vi "Configure ADXL345.vi"(8 "error in":errorcluster, 10 "Port":i8, 11 "FPGA VI Reference":T1) -> (0 "error out":errorcluster, 3 "FPGA VI Reference Out":T1)   [LabVIEW 2014]
uses:
  Controls/FPGA Reference.ctl
  Controls/SPI Configuration Cluster.ctl
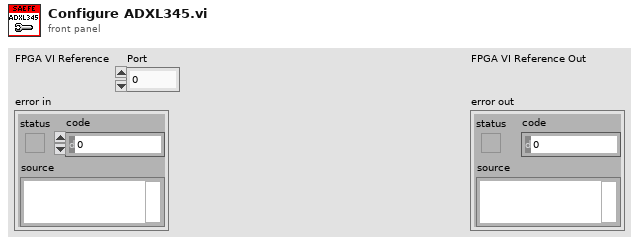
[diagram p1: front panel]
types:
  T1 = typedef "FPGA Reference.ctl" = refnum<k20>
  T2 = typedef "SPI Configuration Cluster.ctl" = cluster{"CS":u8, "Clock Rate (Hz)":dbl, "Clock Mode":u8, "CS Active State":bool}
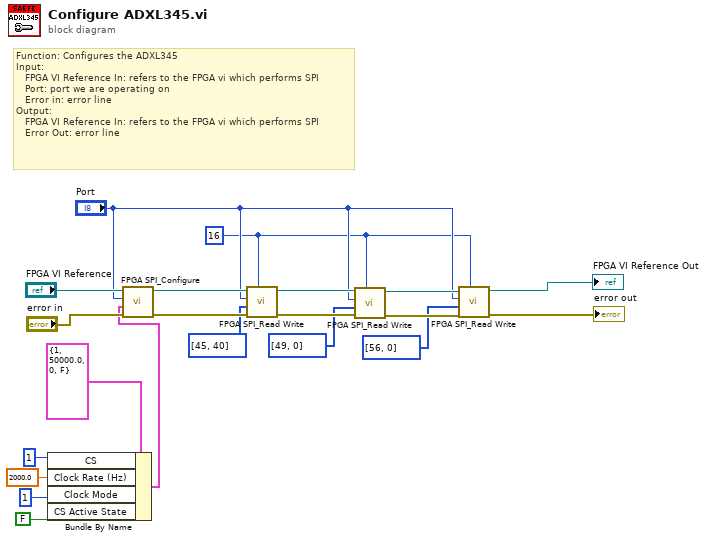
[diagram p0: block diagram]
diagram:
  w3 = u16 16 ("Total Bits")
  # "Function: Configures the ADXL345\nInput:\n   FPGA VI Reference In: refers to the FPGA vi which performs SPI\n   Port: port we are operating on\n   Error in: error line\nOutput:\n   FPGA VI Reference In: refers to the FPGA vi which performs SPI\n   Error Out: error line"
  n1 = Bundle By Name(cluster=T2 {"CS"=1, "Clock Rate (Hz)"=50000.0, "Clock Mode"=0, "CS Active State"=FALSE} ("Configuration Cluster"), "CS"=u8 1, "Clock Rate (Hz)"=2000.0, "Clock Mode"=u8 1, "CS Active State"=FALSE) -> (w16:T2)
  n2 = call "FPGA SPI_Configure.vi"("error in"="error in", "Configuration Cluster"=w16, "Port"="Port", "FPGA VI Reference"="FPGA VI Reference") -> ("error out"=w20:errorcluster, "FPGA VI Reference Out"=w21:T1)  [unwired: 5 in, 1 out]
  n3 = call "FPGA SPI_Read Write.vi"("Total Bits"=w3, "error in"=w20, "Write Data"=u8[] [45, 40], "Port"="Port", "FPGA VI Reference"=w21) -> ("error out"=w9:errorcluster, "FPGA VI Reference Out"=w10:T1)  [unwired: 4 in, 1 out]
  n4 = call "FPGA SPI_Read Write.vi"("Total Bits"=w3, "error in"=w9, "Write Data"=u8[] [49, 0], "Port"="Port", "FPGA VI Reference"=w10) -> ("error out"=w6:errorcluster, "FPGA VI Reference Out"=w7:T1)  [unwired: 4 in, 1 out]
  n5 = call "FPGA SPI_Read Write.vi"("Total Bits"=w3, "error in"=w6, "Write Data"=u8[] [56, 0], "Port"="Port", "FPGA VI Reference"=w7) -> ("error out"=→"error out":errorcluster, "FPGA VI Reference Out"=→"FPGA VI Reference Out":T1)  [unwired: 4 in, 1 out]
